vi "Write Worktable.vi"(8 "error in":errorcluster, 10 "WorkTable in":refnum<class "WorkTable Class.lvclass">, 11 "Potting Procedure in":refnum<class "Potting Procedure.lvclass">) -> (0 "error out":errorcluster, 3 "Potting Procedure out":refnum<class "Potting Procedure.lvclass">)   [LabVIEW 2011, in "Potting Procedure.lvclass"]
uses:
  Potting Procedure.lvclass
  Shared Components/WorkTable Class/WorkTable Class.lvclass
  Potting Procedure.lvclass/Potting Procedure.ctl
  Shared Components/Gantry Class/Gantry Class.lvclass
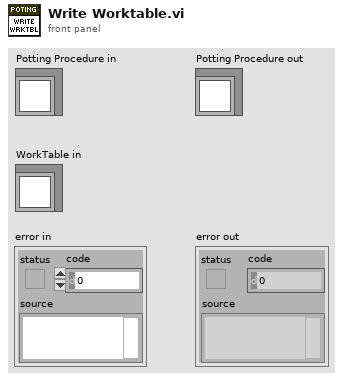
[diagram p1: front panel]
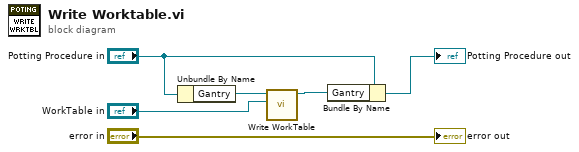
[diagram p0: block diagram]
diagram:
  n1 = Unbundle By Name("Potting Procedure in") -> ("Gantry"=w1:refnum<class "Gantry Class.lvclass">)
  n2 = call-dynamic "Write WorkTable.vi"("WorkTable Class.lvclass"="WorkTable in", "Gantry Class in"=w1) -> ("Gantry Class out"=w4:refnum<class "Gantry Class.lvclass">)  [unwired: 8 in, 1 out]
  n3 = Bundle By Name(cluster="Potting Procedure in", "Gantry"=w4) -> (→"Potting Procedure out":refnum<class "Potting Procedure.lvclass">)
  "error out" <- "error in"
